vi "GetRelativeTimeForGraph.vi"(8 "ErrorIn":errorcluster, 11 "StartTime":timestamp) -> (0 "ErrorOut":errorcluster, 3 "TimeElapsed(s)":dbl)   [LabVIEW 2018]
doc: "This VIs returns the time elapsed since the inputted Start Time\n\nCopyright © 2011 Epimedia, Inc. All Rights Reserved.\n\nThe Epimedia Application Library is Copyright © 2009-2011 Epimedia, Inc. \nAll Rights Reserved. Used under license."
panel:
  # "Copyright © 2011 Epimedia, Inc. All Rights Reserved.\n\nThe Epimedia Application Library is Copyright © 2009-2011 Epimedia, Inc. \nAll Rights Reserved. Used under license."
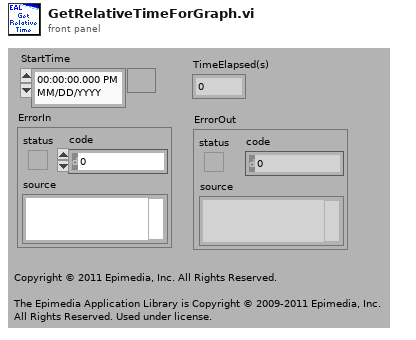
[diagram p1: front panel]
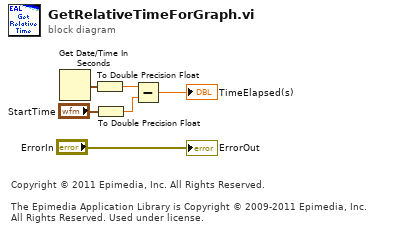
[diagram p0: block diagram]
diagram:
  # "Copyright © 2011 Epimedia, Inc. All Rights Reserved.\n\nThe Epimedia Application Library is Copyright © 2009-2011 Epimedia, Inc. \nAll Rights Reserved. Used under license."
  n1 = Get Date/Time In Seconds() -> (seconds since 1Jan1904=w5:timestamp)
  n2 = To Double Precision Float(number=w5) -> (double precision float=w3:dbl)
  n3 = To Double Precision Float(number="StartTime") -> (double precision float=w2:dbl)
  n4 = Subtract(x=w3, y=w2) -> (x-y=→"TimeElapsed(s)":dbl)
  "ErrorOut" <- "ErrorIn"
